vi "VacLegend.vi"(11 "i ref in":refnum<vi>) -> (3 "i ref out":refnum<vi>)   [LabVIEW 2014, in "Panels.lvlib"]
uses:
  Panels.lvlib
panel:
  out "element 5":u32(colorbox)
  out "element 4":u32(colorbox)
  out "element 3":u32(colorbox)
  out "element 2":u32(colorbox)
  out "element":u32(colorbox)
  # "GUI LEGEND"
  # "Color"
  # "State"
  # "Possible Cause (Det.)"
  # "Possible Cause (Valve)"
  # "Possible Cause (TP)"
  # "No Info Available"
  # "No Link To DIM"
  # "No Link To DIM"
  # "No Link To DIM"
  # "In"
  # "Out"
  # "Open"
  # "Closed"
  # "Run"
  # "Fail"
  # "Stand By - Off"
  # "False"
  # "True"
  # "False"
  # "True"
  # "False"
  # "True"
  # "On"
  # "True"
  # "False"
  # "True"
  # "False"
  # "True"
  # "False"
  # "Warning"
  # "False"
  # "False"
  # "False"
  # "False"
  # "False"
  # "False"
  # "Alarm - Malfunction"
  # "True"
  # "True"
  # "True"
  # "True"
  # "True"
  # "True"
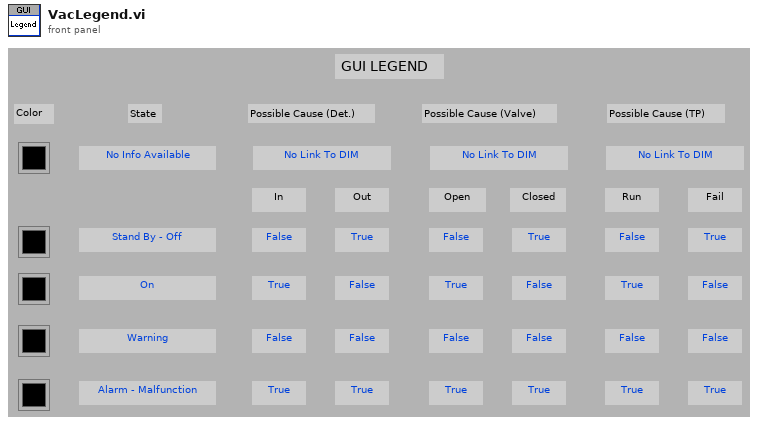
[diagram p1: front panel]
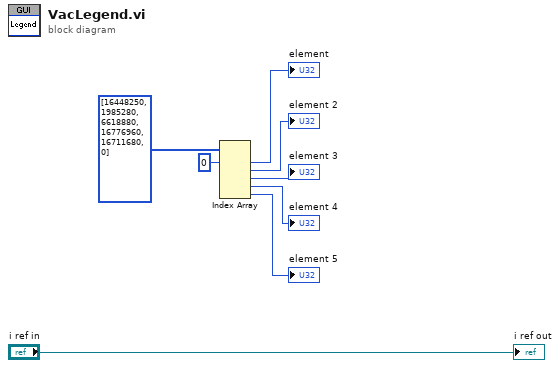
[diagram p0: block diagram]
diagram:
  n1 = Index Array(array=u32[] [16448250, 1985280, 6618880, 16776960, 16711680, 0], index #1=0 ("index")) -> (element #1=→"element":u32, element #2=→"element 2":u32, element #3=→"element 3":u32, element #4=→"element 4":u32, element #5=→"element 5":u32)  [unwired: 4 in]
  "i ref out" <- "i ref in"
